vi "Const load.vi"(2 "send values":bool, 4 "internal force guage (v)":ext format="%.6f", 5 "?":T1 {"lo reset limit" format="%.6f"; "limit" format="%.2f"; "hi reset limit" format="%.6f"; "Prop" format="%.2f"; "Int" format="%.6f"; "set pt" format="%.6f"}) -> (0 "current reset":ext format="%.6f", 1 "Write String":string)   [LabVIEW 2009]
panel:
  # "For stand alone operation, use \"Motor drive globals\" sub VI to set \"Run state\" to on and initial reset value.  Then temporarily wire the while loop inside to run only once."
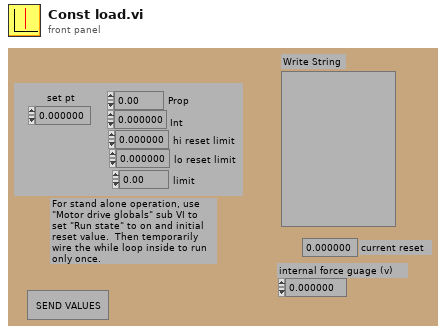
[diagram p1: front panel]
types:
  T1 = cluster{"set pt":ext, "Int":ext, "Prop":ext, "hi reset limit":ext, "limit":ext, "lo reset limit":ext}
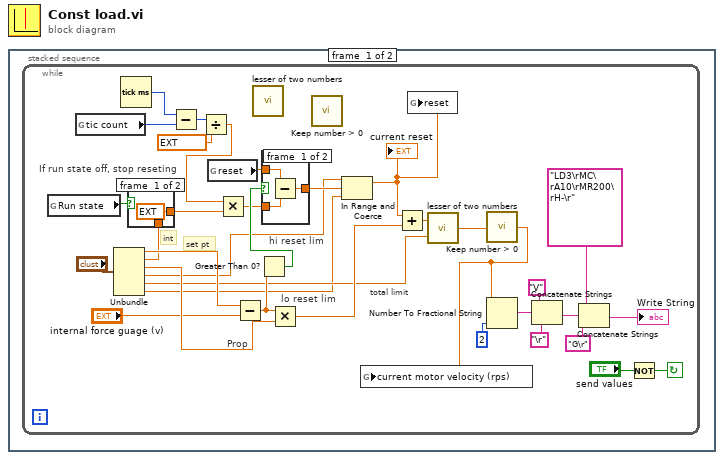
[diagram p0: block diagram]
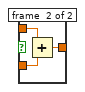
[diagram p3: hidden frame]
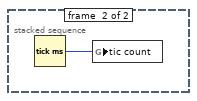
[diagram p4: hidden frame]
diagram:
  n1 = stacked-sequence {
    frame #0 {
      n2 = while {
        stop <- w17 continue-if-true
        # "lo reset lim"
        # "If run state off, stop reseting"
        # "total limit"
        # "int"
        # "hi reset lim"
        # "set pt"
        # "Prop"
        n3 = global read "Motor drive globals" "Run state"() -> (w21:bool)
        n4 = global read "Motor drive globals" "tic count"() -> (w27:u32)
        n5 = Unbundle("?") -> ("set pt"=w29:ext, "Int"=w19:ext, "Prop"=w28:ext, "hi reset limit"=w3:ext, "limit"=w23:ext, "lo reset limit"=w2:ext)
        n6 = Tick Count (ms)() -> (millisecond timer value=w26:u32)
        n7 = case shown="False" w21 {
          tunnel: [ext 0.0 w37] -> w20
          tunnel: w19 -> [_ w37]
          frame #0 {
          }
          frame #1 {
          }
        }
        n8 = Subtract(x=w26, y=w27) -> (x-y=w32:u32)
        n9 = Divide(x=w32, y=ext 1000.0) -> (x/y=w25:ext)
        n10 = global read "Motor drive globals" "reset"() -> (w5:ext)
        n11 = Multiply(x=w25, y=w20) -> (x*y=w31:ext)
        n12 = Subtract(x=w29, y="internal force guage (v)") -> (x-y=w35:ext)
        n13 = call "lesser of two numbers"() -> ()  [unwired: 2 in, 1 out]
        n14 = Greater Than 0?(x=w35) -> (x > 0?=w34:bool)
        n15 = case shown="True" w34 {
          tunnel: w5 -> [w39 w43]
          tunnel: w31 -> [w40 w42]
          tunnel: [w38 w41] -> w4
          frame #0 {
            n16 = Subtract(x=w39, y=w40) -> (x-y=w38:ext)
          }
          frame #1 {
            n17 = Add(x=w43, y=w42) -> (x+y=w41:ext)
          }
        }
        n18 = Multiply(x=w35, y=w28) -> (x*y=w24:ext)
        n19 = call "Keep number > 0"() -> ()  [unwired: 1 in, 1 out]
        n20 = In Range and Coerce(upper limit=w3, x=w4, lower limit=w2) -> (coerced(x)=w1:ext)  [unwired: 1 out]
        "current reset" <- w1
        n21 = Add(x=w1, y=w24) -> (x+y=w22:ext)
        n22 = global write "Motor drive globals" "reset"(w1) -> ()
        n23 = call "lesser of two numbers"("y"=w23, "x"=w22) -> ("lesser value"=w9:ext)
        n24 = call "Keep number > 0"("In"=w9) -> ("Out"=w6:ext)
        n25 = global write "Motor drive globals" "current motor velocity (rps)"(w6) -> ()
        n26 = Number To Fractional String(number=w6, precision (6)=2) -> (F-format string=w15:string)  [unwired: 2 in]
        n27 = Concatenate Strings("V", w15, "\r") -> (w12:string)
        n28 = Concatenate Strings("LD3\rMC\rA10\rMR200\rH-\r", w12, "G\r") -> (→"Write String":string)
        n29 = Not(x="send values") -> (.not. x?=w17:bool)
      }
    }
    frame #1 {
      n30 = Tick Count (ms)() -> (millisecond timer value=w44:u32)
      n31 = global write "Motor drive globals" "tic count"(w44) -> ()
    }
  }
